vi "Get Image Data.vi"(8 "error in (no error)":errorcluster caption="错误输入（无错误）", 11 "Gif Image 输入":refnum<class "Gif Image.lvclass"> caption="DNL_LabVIEW Object in") -> (0 "error out":errorcluster caption="错误输出", 3 "Gif Image 输出":refnum<class "Gif Image.lvclass"> caption="DNL_LabVIEW Object out")   [LabVIEW 2011, in "Gif Image.lvclass"]
uses:
  Gif Image.lvclass
  Control/Image Descriptor.ctl
panel:
  out "Index Array":i32[](array[numeric])
  in  "Image Descriptor":T1
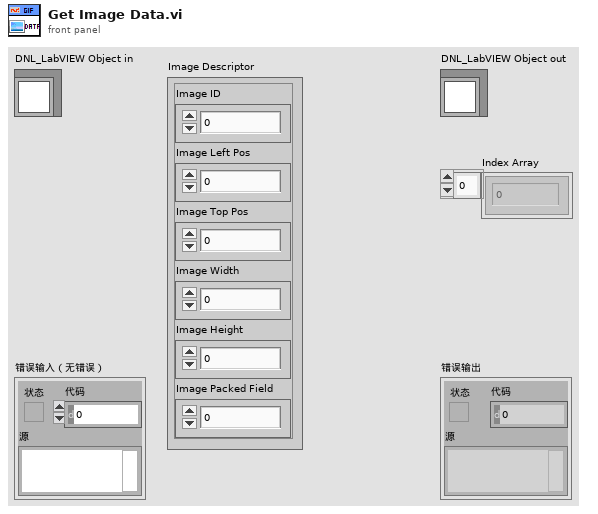
[diagram p1: front panel]
types:
  T1 = typedef "Gif Image.lvclass/Image Descriptor.ctl" = cluster{"Image ID":u8, "Image Left Pos":u16, "Image Top Pos":u16, "Image Width":u16, "Image Height":u16, "Image Packed Field":u8}
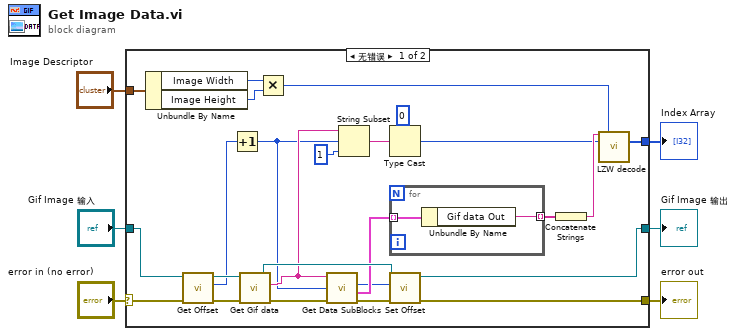
[diagram p0: block diagram]
diagram:
  n1 = case shown="无错误" "error in (no error)" {
    selector: "error in (no error)" -> [w9 w35]
    tunnel: [w8 w35] -> w5
    tunnel: [w22 w34] -> w3
    tunnel: "Gif Image 输入" -> [w26 w34]
    tunnel: "Image Descriptor" -> [w31 _]
    tunnel: [w11 _] -> w1
    frame No Error {
      n2 = Unbundle By Name(w31) -> ("Image Width"=w29:u16, "Image Height"=w30:u16)
      n3 = call "Get Offset.vi"("error in (no error)"=w9, "Gif Image输入"=w26) -> ("error out"=w27:errorcluster, "Offset"=w25:i32, "Gif Image输出"=w28:refnum<class "Gif Image.lvclass">)  [unwired: 7 in]
      n4 = Increment(x=w25) -> (x+1=w16:i32)
      n5 = call "Get Gif data.vi"("error in (no error)"=w27, "Gif Image输入"=w28) -> ("error out"=w24:errorcluster, "Gif data"=w17:string, "Gif Image输出"=w23:refnum<class "Gif Image.lvclass">)  [unwired: 7 in]
      n6 = Multiply(x=w29, y=w30) -> (x*y=w18:u16)
      n7 = call "Get Data SubBlocks.vi"("错误输入"=w24, "Offset In"=w16, "Gif data in"=w17) -> ("错误输出"=w10:errorcluster, "Data Blocks"=w21:cluster{"Len":u8, "Gif data Out":string}[], "Offset Out"=w7:i32)  [unwired: 5 in, 1 out]
      n8 = String Subset(string=w17, offset (0)=w16, length (rest)=1 ("长度（剩余）")) -> (substring=w14:string)
      n9 = Type Cast(type=u8 0, x=w14) -> (*(type *) &x=w12:u8)
      n10 = for {
        tunnel: w21 -> [w33] mode=indexing
        tunnel: [w32] -> w20 mode=indexing
        n11 = Unbundle By Name(w33) -> ("Gif data Out"=w32:string)
      }
      n12 = call "Set Offset.vi"("error in (no error)"=w10, "Offset"=w7, "Gif Image输入"=w23) -> ("error out"=w8:errorcluster, "Gif Image输出"=w22:refnum<class "Gif Image.lvclass">)  [unwired: 7 in]
      n13 = Concatenate Strings(w20) -> (w19:string)
      n14 = call "LZW decode.vi"("data"=w19, "expected data size"=w18, "NumberOfStartBits"=w12) -> ("decoded data"=w11:i32[])  [unwired: 11 in, 1 out]
    }
    frame Error {
    }
  }
  "error out" <- w5
  "Gif Image 输出" <- w3
  "Index Array" <- w1
